vi "BundleMagic TOP.vi"(6 "Mouse Position":cluster{"Left":i32, "Top":i32}, 8 "User VI Ref":refnum<vi>, 9 "Menu Item Tag Suffix":string, 10 "Remaining Items":refnum<vi>[](array[refnum]), 11 "Affected Items":T1) -> (0 "Fail transaction?":bool)   [LabVIEW 2023]
doc: "Note: This plugin utilizes the scripting code originally written by wiebe@CARYA and posted as a Quick Drop Keyboard Shortcut here:\n\nhttps://decibel.ni.com/content/docs/DOC-37156"
panel:
  # "All controls on this panel except \"Affected Items\" have been locked to prevent accidental edits. Changing the control names or types, other than the elements of the \"Affected Items\" cluster will make the VI unusable as a menu plugin.\n\nSee Context Help for each control for details about its use."
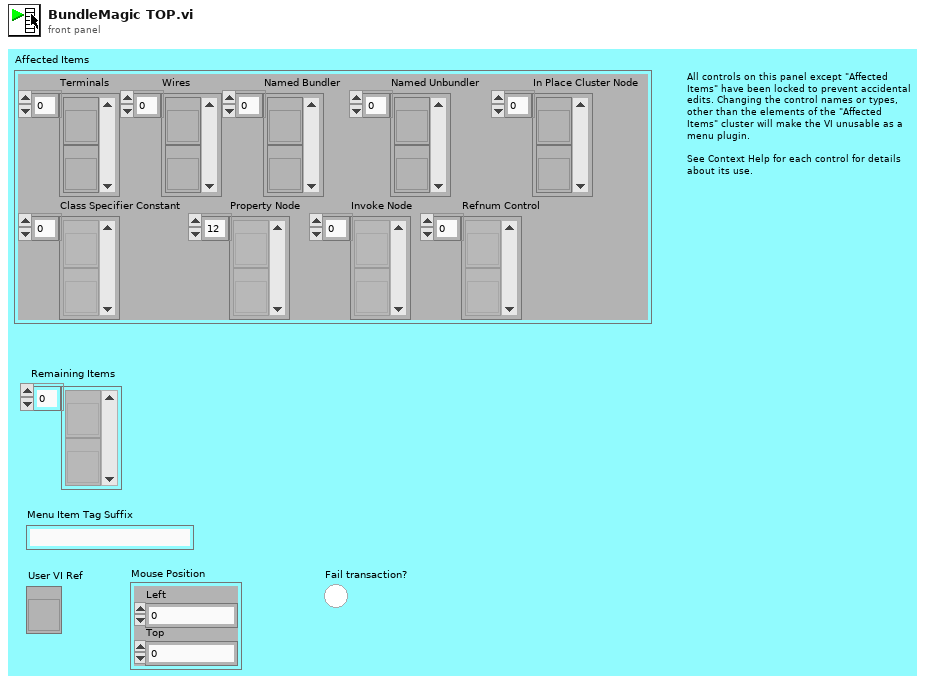
[diagram p1: front panel]
types:
  T1 = cluster{"Terminals":refnum<vi>[], "Wires":refnum<vi>[], "Named Bundler":refnum<vi>[], "Named Unbundler":refnum<vi>[], "In Place Cluster Node":refnum<vi>[], "Class Specifier Constant":refnum<vi>[], "Property Node":refnum<vi>[], "Invoke Node":refnum<vi>[], "Refnum Control":refnum<vi>[]}
  T2 = enum16{"[NONE]", "Wire Bundle", "Wire Unbundle", "Terminal Unbundle", "Terminal Bundle", "Bundler Move Up", "Bundler Move Down", "Bundler Insert", "Bundler Remove", "Bundler Remove Unwired", "Bundler Rearrange", "In Place Insert", "In Place Remove", "In Place Remove Unwired", "In Place Rearrange", "Wire Properties", "Wire Method", "Terminal Properties", "Terminal Method", "Property Move Up", "Property Move Down", "Properties Insert", "Properties Remove", "Properties Remove Unwired", "Properties Rearrange", "Method Change", "Class For Constant", "Class For Control", "Class For Node", "Class Name to Clipboard"}
  T3 = enum16{"None", "Cluster", "Property", "Method", "Class"}
  T4 = cluster{"Element Label":string, "Nest Chain":string[], "Is Cluster?":bool, "Data Type":variant, "Bundler Label":string, "Disabled":bool, "Unwired":bool, "Tree Tag":string}[]
  T5 = cluster{"Tag":string, "Read":bool, "Write":bool, "New":bool}[]
  T6 = cluster{"Label":string, "Tag":string, "Property Type":enum16{"Unknown", "Base", "Scripting", "Private", "Deprecated", "None", "Divider"}, "Indent":u16, "Can Read?":bool, "Can Write?":bool, "Is Read?":bool, "Is Write?":bool, "Inactive Parent?":bool, "Unwired?":bool}[]
  T7 = cluster{"Class Info":cluster{"Unique ID string":string, "Parent ID string":string, "Class Name (unlocalized)":string, "Class Name (localized)":string}, "Class Heirarchy":string, "Class Type":enum16{"Unknown", "Base", "Scripting", "Private", "Deprecated", "None", "Divider"}, "Indent":u32}[]
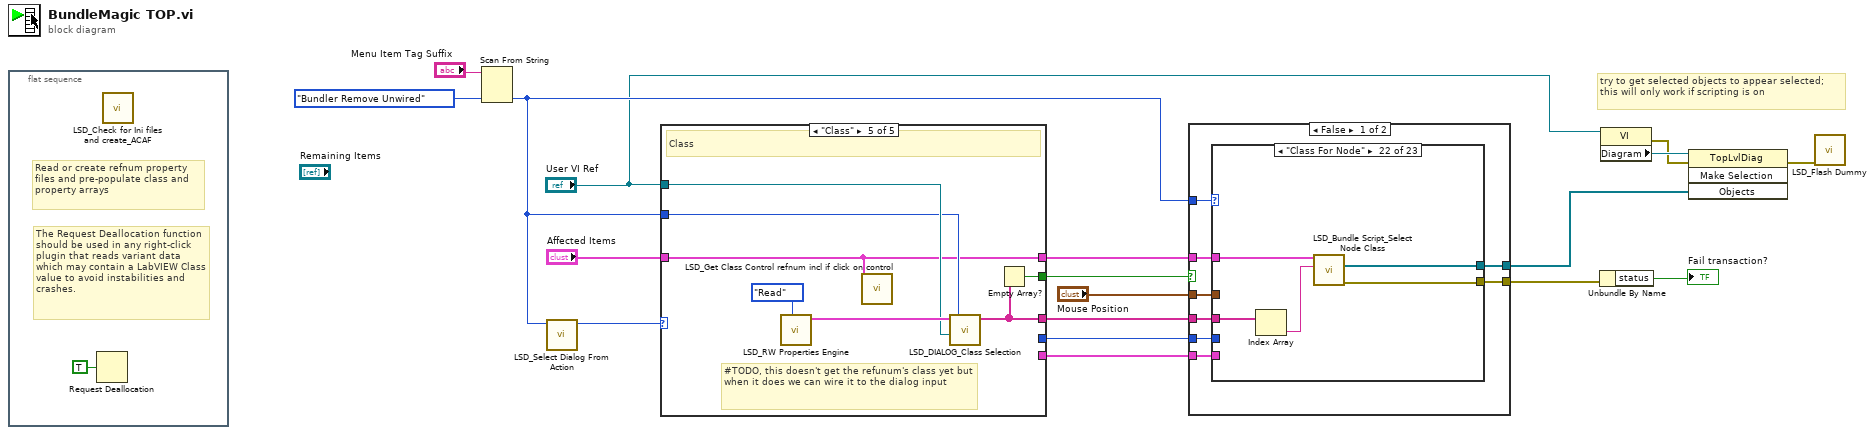
[diagram p0: block diagram]
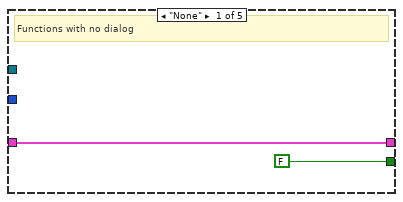
[diagram p2: hidden frame]
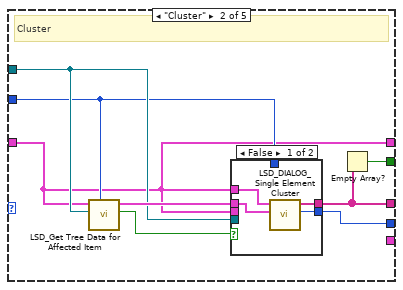
[diagram p3: hidden frame]
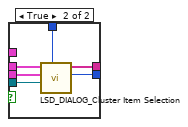
[diagram p4: hidden frame]
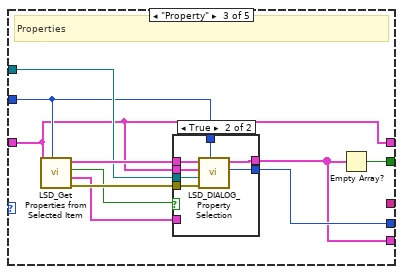
[diagram p5: hidden frame]
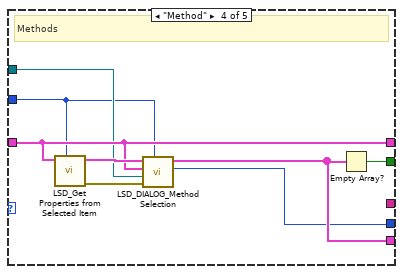
[diagram p7: hidden frame]
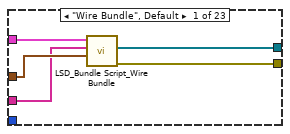
[diagram p8: hidden frame]
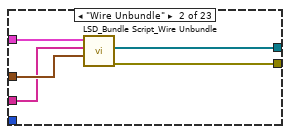
[diagram p9: hidden frame]
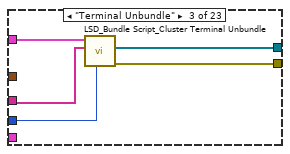
[diagram p10: hidden frame]
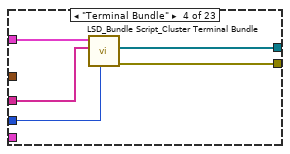
[diagram p11: hidden frame]
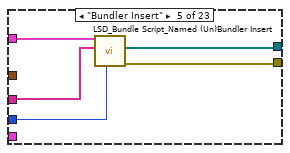
[diagram p12: hidden frame]
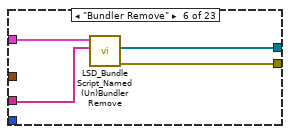
[diagram p13: hidden frame]
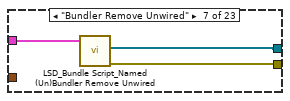
[diagram p14: hidden frame]
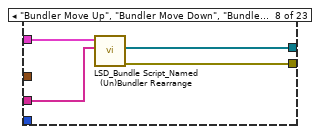
[diagram p15: hidden frame]
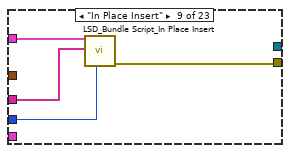
[diagram p16: hidden frame]
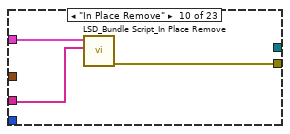
[diagram p17: hidden frame]
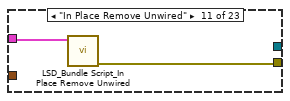
[diagram p18: hidden frame]
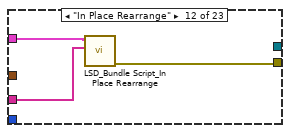
[diagram p19: hidden frame]
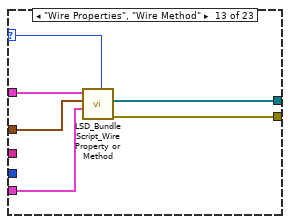
[diagram p20: hidden frame]
diagram:
  # "try to get selected objects to appear selected; this will only work if scripting is on"
  n1 = flat-sequence {
    frame #0 {
      # "The Request Deallocation function should be used in any right-click plugin that reads variant data which may contain a LabVIEW Class value to avoid instabilities and crashes."
      # "Read or create refnum property files and pre-populate class and property arrays"
      n2 = Request Deallocation(TRUE ("flag")) -> ()
      n3 = call <resource>:"LSD_Check for Ini files and create_ACAF.vi"() -> ()  [unwired: 11 in, 1 out]
    }
  }
  n4 = Scan From String(input string="Menu Item Tag Suffix", default 1=T2."Bundler Remove Unwired" ("Action")) -> (output 1=w4:T2)  [unwired: 3 in, 3 out]
  n5 = call <resource>:"LSD_Select Dialog From Action.vi"("Action"=w4) -> ("Dialog Selection"=w5:T3)  [unwired: 10 in]
  n6 = case shown="\"Class\"" w5 {
    tunnel: [_ w27 w47 w60 _] -> w15
    tunnel: "User VI Ref" -> [_ w28 w48 w64 w71]
    tunnel: [_ w26 _ _ w69] -> w14
    tunnel: [w21 w22 w41 w65 w67] -> w11
    tunnel: "Affected Items" -> [w21 w22 w41 w65 w67]
    tunnel: [_ _ w42 w62 _] -> w10
    tunnel: [FALSE ("empty?") w25 w46 w63 w70] -> w9
    tunnel: w4 -> [_ w24 w45 w61 w68]
    frame "None" {
      # "Functions with no dialog"
    }
    frame "Cluster" {
      # "Cluster"
      n7 = call <resource>:"LSD_Get Tree Data for Affected Item.vi"("Action"=w24, "User VI Ref"=w28, "Affected Items"=w22) -> ("Use Dialog?"=w23:bool, "Elements Array"=w29:T4)  [unwired: 7 in]
      n8 = case shown="False" w23 {
        tunnel: w29 -> [w33 w39]
        tunnel: w28 -> [_ w38]
        tunnel: w22 -> [_ w37]
        tunnel: [w30 w36] -> w27
        tunnel: [w31 w35] -> w26
        tunnel: w24 -> [_ w34]
        tunnel: w22 -> [w32 _]
        frame False {
          n9 = call <resource>:"LSD_DIALOG_Single Element Cluster.vi"("Display Items"=w33, "Affected Items"=w32) -> ("Placement Out"=w30:enum32{"Choice 1", "Choice 2"}, "Selected Items (tags)"=w31:string[])  [unwired: 8 in]
        }
        frame True {
          n10 = call <resource>:"LSD_DIALOG_Cluster Item Selection.vi"("Action"=w34, "User VI Ref"=w38, "Affected Items"=w37, "Display Items"=w39) -> ("Action Choice Out"=w36:enum32{"Choice 1", "Choice 2"}, "Selected Items (tags)"=w35:string[])  [unwired: 5 in, 1 out]
        }
      }
      n11 = Empty Array?(array=w26) -> (empty?=w25:bool)
    }
    frame "Property" {
      # "Properties"
      n12 = call <resource>:"LSD_Get Properties from Selected Item.vi"("Action"=w45, "Affected Items"=w41) -> ("Error Out"=w44:errorcluster, "Property Array Out"=w40:T5, "Use Dialog?"=w43:bool, "Properties for Tree Out"=w49:T6)  [unwired: 6 in]
      n13 = case shown="True" w43 {
        tunnel: w49 -> [_ w58]
        tunnel: w41 -> [_ w57]
        tunnel: w48 -> [_ w56]
        tunnel: [w51 w55] -> w47
        tunnel: [w50 w52] -> w42
        tunnel: w45 -> [w51 w54]
        tunnel: w44 -> [_ w53]
        tunnel: w40 -> [w50 _]
        frame False {
        }
        frame True {
          n14 = call <resource>:"LSD_DIALOG_Property Selection.vi"("Action"=w54, "Error In"=w53, "User VI Ref"=w56, "Affected Items"=w57, "Properties for Tree In"=w58) -> ("Placement Out"=w55:enum32{"Choice 1", "Choice 2"}, "Property Array Out"=w52:T5)  [unwired: 4 in, 1 out]
        }
      }
      n15 = Empty Array?(array=w42) -> (empty?=w46:bool)
    }
    frame "Method" {
      # "Methods"
      n16 = call <resource>:"LSD_Get Properties from Selected Item.vi"("Action"=w61, "Affected Items"=w65) -> ("Error Out"=w59:errorcluster, "Properties for Tree Out"=w66:T6)  [unwired: 6 in, 2 out]
      n17 = call <resource>:"LSD_DIALOG_Method Selection.vi"("Action"=w61, "Error In"=w59, "User VI Ref"=w64, "Affected Items"=w65, "Methods for Tree In"=w66) -> ("Placement Out"=w60:enum32{"Choice 1", "Choice 2"}, "Method Array Out"=w62:T5)  [unwired: 4 in, 1 out]
      n18 = Empty Array?(array=w62) -> (empty?=w63:bool)
    }
    frame "Class" {
      # "#TODO, this doesn't get the refunum's class yet but when it does we can wire it to the dialog input"
      # "Class"
      n19 = call <resource>:"LSD_RW Properties Engine.vi"("File Action [Read]"=enum16{"Read", "Write"}."Read") -> ("Classes Out"=w73:T7)  [unwired: 5 in, 5 out]
      n20 = call <resource>:"LSD_Get Class Control refnum incl if click on control.vi"("Affected Items"=w67) -> ()  [unwired: 9 in, 2 out]
      n21 = call <resource>:"LSD_DIALOG_Class Selection.vi"("Action"=w68, "User VI Ref"=w71, "Classes"=w73) -> ("Unique ID of Selected Item"=w69:string[])  [unwired: 7 in, 1 out]
      n22 = Empty Array?(array=w69) -> (empty?=w70:bool)
    }
  }
  n23 = case shown="False" w9 {
    tunnel: w11 -> [w81 _]
    tunnel: "Mouse Position" -> [w80 _]
    tunnel: w14 -> [w79 _]
    tunnel: w15 -> [w78 _]
    tunnel: w4 -> [w77 _]
    tunnel: w10 -> [w76 _]
    tunnel: [w75 _] -> w8
    tunnel: [w74 refnum<vi>[] [] ("Objects")] -> w3
    frame False {
      n24 = case shown="\"Class For Node\"" w77 {
        selector: w77 -> [_ _ _ _ _ _ _ _ _ _ _ _ w132 w138 _ _ _ _ _ _ _ _ _]
        tunnel: w81 -> [w86 w91 w96 w101 w106 w110 w113 w117 w121 w124 w126 w129 w135 w141 w146 w150 w153 w157 w161 w166 w170 w175 w178]
        tunnel: w80 -> [w85 w90 _ _ _ _ _ _ _ _ _ _ w134 _ _ _ _ _ _ _ _ _ _]
        tunnel: w79 -> [w84 w89 w94 w99 w104 w109 _ w116 w119 w123 _ w128 _ _ _ _ _ _ _ w165 w171 w176 _]
        tunnel: w78 -> [_ _ w95 w100 w105 _ _ _ w120 _ _ _ _ w139 w144 _ _ _ _ _ _ _ _]
        tunnel: w76 -> [_ _ _ _ _ _ _ _ _ _ _ _ w133 w140 w145 w147 _ w156 w160 _ _ _ _]
        tunnel: [w83 w88 w93 w98 w103 w108 w112 w115 w118 w122 w125 w127 w131 w137 w143 w149 w151 w155 w159 w163 w168 w172 w177] -> w75
        tunnel: [w82 w87 w92 w97 w102 w107 w111 w114 _ _ _ _ w130 w136 w142 w148 w152 w154 w158 w162 w167 w174 _] -> w74
        frame "Wire Bundle", Default {
          n25 = call <resource>:"LSD_Bundle Script_Wire Bundle.vi"("Mouse Position"=w85, "Selected Items Tags"=w84, "Affected Items"=w86) -> ("error out"=w83:errorcluster, "Objects"=w82:refnum<vi>[])  [unwired: 7 in]
        }
        frame "Wire Unbundle" {
          n26 = call <resource>:"LSD_Bundle Script_Wire Unbundle.vi"("Mouse Position"=w90, "Selected Items Tags"=w89, "Affected Items"=w91) -> ("error out"=w88:errorcluster, "Objects"=w87:refnum<vi>[])  [unwired: 7 in]
        }
        frame "Terminal Unbundle" {
          n27 = call <resource>:"LSD_Bundle Script_Cluster Terminal Unbundle.vi"("Object Placement"=w95, "Selected Items Tags"=w94, "Affected Items"=w96) -> ("error out"=w93:errorcluster, "Objects"=w92:refnum<vi>[])  [unwired: 7 in]
        }
        frame "Terminal Bundle" {
          n28 = call <resource>:"LSD_Bundle Script_Cluster Terminal Bundle.vi"("Object Placement"=w100, "Selected Items Tags"=w99, "Affected Items"=w101) -> ("error out"=w98:errorcluster, "Objects"=w97:refnum<vi>[])  [unwired: 7 in]
        }
        frame "Bundler Insert" {
          n29 = call <resource>:"LSD_Bundle Script_Named (Un)Bundler Insert.vi"("Dialog Choice"=w105, "Selected Items (tags)"=w104, "Affected Items"=w106) -> ("error out"=w103:errorcluster, "Objects"=w102:refnum<vi>[])  [unwired: 7 in]
        }
        frame "Bundler Remove" {
          n30 = call <resource>:"LSD_Bundle Script_Named (Un)Bundler Remove.vi"("Selected Items (tags)"=w109, "Affected Items"=w110) -> ("error out"=w108:errorcluster, "Objects"=w107:refnum<vi>[])  [unwired: 8 in]
        }
        frame "Bundler Remove Unwired" {
          n31 = call <resource>:"LSD_Bundle Script_Named (Un)Bundler Remove Unwired.vi"("Affected Items"=w113) -> ("error out"=w112:errorcluster, "Objects"=w111:refnum<vi>[])  [unwired: 9 in]
        }
        frame "Bundler Move Up", "Bundler Move Down", "Bundler Rearrange" {
          n32 = call <resource>:"LSD_Bundle Script_Named (Un)Bundler Rearrange.vi"("Displayed Items"=w116, "Affected Items"=w117) -> ("error out"=w115:errorcluster, "Objects"=w114:refnum<vi>[])  [unwired: 8 in]
        }
        frame "In Place Insert" {
          n33 = call <resource>:"LSD_Bundle Script_In Place Insert.vi"("Action Choice In"=w120, "Selected Items Tags"=w119, "Affected Items"=w121) -> ("error out"=w118:errorcluster)  [unwired: 8 in]
        }
        frame "In Place Remove" {
          n34 = call <resource>:"LSD_Bundle Script_In Place Remove.vi"("Selected Items Tags"=w123, "Affected Items"=w124) -> ("error out"=w122:errorcluster)  [unwired: 9 in]
        }
        frame "In Place Remove Unwired" {
          n35 = call <resource>:"LSD_Bundle Script_In Place Remove Unwired.vi"("Affected Items"=w126) -> ("error out"=w125:errorcluster)  [unwired: 10 in]
        }
        frame "In Place Rearrange" {
          n36 = call <resource>:"LSD_Bundle Script_In Place Rearrange.vi"("Displayed Items"=w128, "Affected Items"=w129) -> ("error out"=w127:errorcluster)  [unwired: 9 in]
        }
        frame "Wire Properties", "Wire Method" {
          n37 = call <resource>:"LSD_Bundle Script_Wire Property or Method.vi"("Action"=w132, "Property Array"=w133, "Mouse Position"=w134, "Affected Items"=w135) -> ("error out"=w131:errorcluster, "Objects"=w130:refnum<vi>[])  [unwired: 6 in]
        }
        frame "Terminal Properties", "Terminal Method" {
          n38 = call <resource>:"LSD_Bundle Script_Terminal Property or Method.vi"("Object Placement"=w139, "Action"=w138, "Property Array"=w140, "Affected Items"=w141) -> ("error out"=w137:errorcluster, "Objects"=w136:refnum<vi>[])  [unwired: 6 in]
        }
        frame "Properties Insert" {
          n39 = call <resource>:"LSD_Bundle Script_Property Insert.vi"("Dialog Choice"=w144, "Property Array"=w145, "Affected Items"=w146) -> ("error out"=w143:errorcluster, "Objects"=w142:refnum<vi>[])  [unwired: 7 in]
        }
        frame "Properties Remove" {
          n40 = call <resource>:"LSD_Bundle Script_Properties Remove.vi"("Property Array"=w147, "Affected Items"=w150) -> ("error out"=w149:errorcluster, "Objects"=w148:refnum<vi>[])  [unwired: 8 in]
        }
        frame "Properties Remove Unwired" {
          n41 = call <resource>:"LSD_Bundle Script_Properties Remove Unwired.vi"("Affected Items 2"=w153) -> ("error out"=w151:errorcluster, "Objects"=w152:refnum<vi>[])  [unwired: 9 in]
        }
        frame "Property Move Up", "Property Move Down", "Properties Rearrange" {
          n42 = call <resource>:"LSD_Bundle Script_Properties Rearrange.vi"("Property Array"=w156, "Affected Items"=w157) -> ("error out"=w155:errorcluster, "Objects"=w154:refnum<vi>[])  [unwired: 8 in]
        }
        frame "Method Change" {
          n43 = call <resource>:"LSD_Bundle Script_Invoke Node Method Change.vi"("Property Array"=w160, "Affected Items"=w161) -> ("error out"=w159:errorcluster, "Objects"=w158:refnum<vi>[])  [unwired: 8 in]
        }
        frame "Class For Constant" {
          n44 = Index Array(array=w165) -> (element=w164:string)  [unwired: 1 in]
          n45 = call <resource>:"LSD_Bundle Script_Select Constant Class.vi"("ID String"=w164, "Affected Items"=w166) -> ("error out"=w163:errorcluster, "Objects"=w162:refnum<vi>[])  [unwired: 8 in]
        }
        frame "Class For Control" {
          n46 = Index Array(array=w171) -> (element=w169:string)  [unwired: 1 in]
          n47 = call <resource>:"LSD_Bundle Script_Select Control Class.vi"("ID String"=w169, "Affected Items"=w170) -> ("error out"=w168:errorcluster, "Objects"=w167:refnum<vi>[])  [unwired: 8 in]
        }
        frame "Class For Node" {
          n48 = Index Array(array=w176) -> (element=w173:string)  [unwired: 1 in]
          n49 = call <resource>:"LSD_Bundle Script_Select Node Class.vi"("ID String"=w173, "Affected Items"=w175) -> ("error out"=w172:errorcluster, "Objects"=w174:refnum<vi>[])  [unwired: 8 in]
        }
        frame "Class Name to Clipboard" {
          n50 = call <resource>:"LSD_Bundle Script_Class Name to Clipboard.vi"("Affected Items"=w178) -> ("error out"=w177:errorcluster)  [unwired: 10 in]
        }
      }
    }
    frame True {
    }
  }
  n51 = Unbundle By Name(w8) -> ("status"=→"Fail transaction?":bool)
  n52 = property class="VI"(reference="User VI Ref") -> (error out=w17:errorcluster, "Diagram"=w18:refnum<vi>)  [unwired: 1 in, 1 out]
  n53 = invoke class="TopLvlDiag" method="Make Selection"(reference=w18, error in=w17, "Objects"=w3) -> (error out=w13:errorcluster)  [unwired: 1 in, 3 out]
  n54 = call <resource>:"LSD_Flash Dummy.vi"("Error In"=w13) -> ()  [unwired: 10 in, 1 out]
